vi "TC.vi"(10 "Target Temperature":dbl format="%#.1f °C", 11 "Temperature":dbl format="%#.1f °C") -> ()   [LabVIEW 2013]
panel:
  out "Heating":u8(slide) caption="%" scale=0.0..100.0
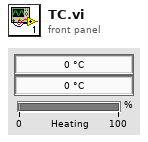
[diagram p1: front panel]
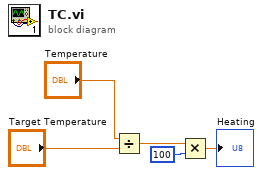
[diagram p0: block diagram]
diagram:
  n1 = Divide(x="Temperature", y="Target Temperature") -> (x/y=w3:dbl)
  n2 = Multiply(x=w3, y=100) -> (x*y=→"Heating":dbl)
